vi "Destroy.vi"(8 "error in (no error)":errorcluster, 11 "MCListbox with Checkboxes.lvclass":refnum<class "MCListbox with Checkboxes.lvclass">) -> (0 "error out":errorcluster)   [LabVIEW 2016, in "MCListbox with Checkboxes.lvclass"]
uses:
  MCListbox with Checkboxes.lvclass
  MCListbox with Checkboxes.lvclass/MCListbox with Checkboxes.ctl
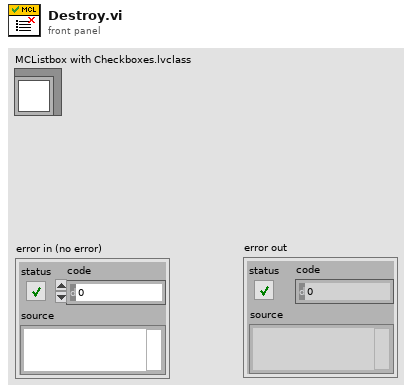
[diagram p1: front panel]
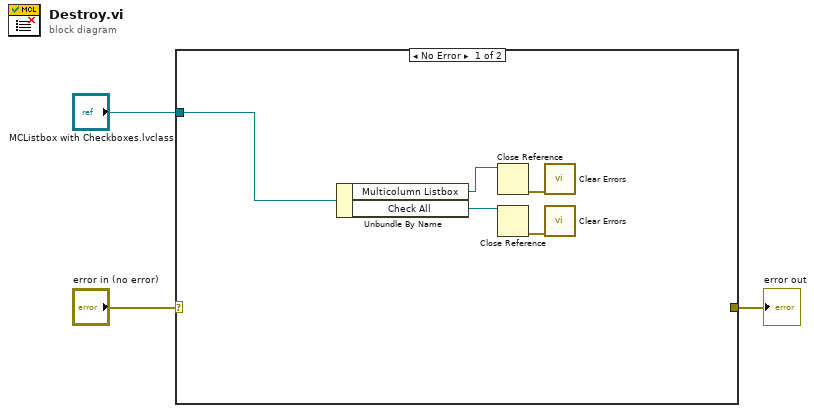
[diagram p0: block diagram]
diagram:
  n1 = case shown="No Error" "error in (no error)" {
    selector: "error in (no error)" -> [_ w9]
    tunnel: "MCListbox with Checkboxes.lvclass" -> [w8 _]
    tunnel: [_ w9] -> w1
    frame No Error {
      n2 = Unbundle By Name(w8) -> ("Multicolumn Listbox"=w7:refnum<vi>, "Check All"=w4:refnum<vi>)
      n3 = Close Reference(reference=w7) -> (error out=w6:errorcluster)  [unwired: 1 in]
      n4 = Close Reference(reference=w4) -> (error out=w5:errorcluster)  [unwired: 1 in]
      n5 = call <vilib>:"Clear Errors.vi"("error in (no error)"=w6) -> ()  [unwired: 5 in, 2 out]
      n6 = call <vilib>:"Clear Errors.vi"("error in (no error)"=w5) -> ()  [unwired: 5 in, 2 out]
    }
    frame Error {
    }
  }
  "error out" <- w1
